vi "FaulhaberCommunication.vi"(7 "axis-optional-1":i16=-1, 8 "error in (no error)":errorcluster, 9 "Argument-optional":dbl=nan, 10 "Befehl":string="GAC", 11 "VISA resource name":refnum<visa-resource-name>="COM10") -> (0 "error out":errorcluster={"status"=FALSE, "code"=1073676293, "source"="VISA Read in FaulhaberCommunication.vi->Faulhaber_Standalone.vi"}, 1 "return":dbl, 2 "return":string="5000\r\n", 3 "VISA resource name out":refnum<visa-resource-name>="COM10")   [LabVIEW 2011]
uses:
  <vilib>/Instr/_visa.llb/VISA Flush IO Buffer Mask.ctl
panel:
  out "return count":u32=6
  in  "Array":T1(array[cluster])
  out "expect return":T2(ring)=enum."somethingelse16"
  out "to send unsigned byte array":u8[](array[numeric])=[71, 65, 67, 13] format="%02x"
  out "send":u32=4
  # "send ist CR\nZwischen befehl und Argument kein leerzeichen\nArgument bis I32\nantwort ist CR-LF"
  # "Gibt binär return:"
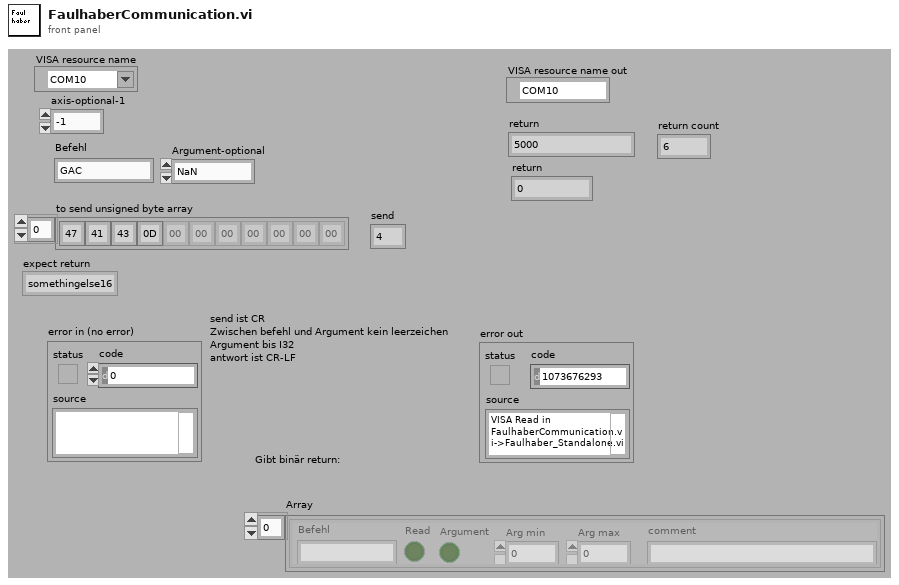
[diagram p1: front panel]
types:
  T1 = cluster{"Befehl":string, "Read":bool, "Arg min":dbl, "Arg max":dbl, "Argument":bool, "comment":string}[]
  T2 = enum8{"none", "program32", "program16", "data32", "data16", "eprom32", "eprom16", "somethingelse32", "somethingelse16"}
  T3 = typedef "VISA Flush IO Buffer Mask.ctl" = u16
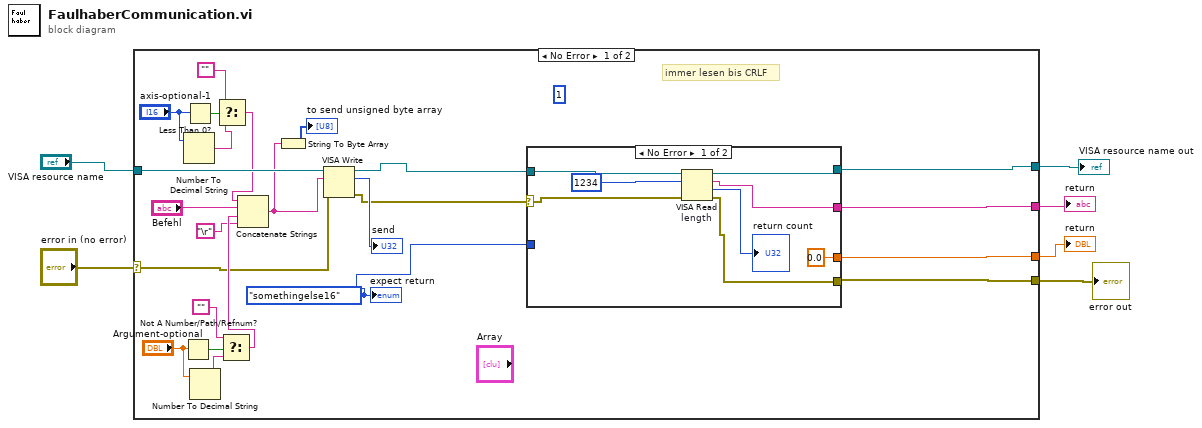
[diagram p0: block diagram]
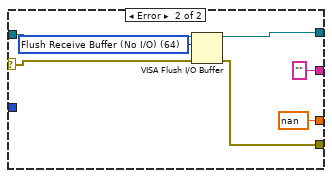
[diagram p2: hidden frame]
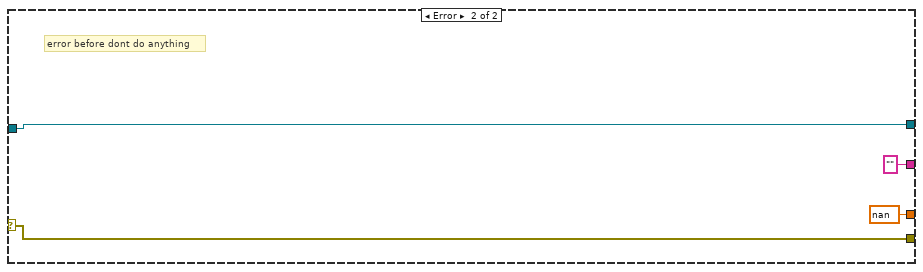
[diagram p3: hidden frame]
diagram:
  n1 = case shown="No Error" "error in (no error)" {
    selector: "error in (no error)" -> [w12 w48]
    tunnel: "VISA resource name" -> [w30 w49]
    tunnel: [w28 w49] -> w5
    tunnel: [w27 w48] -> w4
    tunnel: [w26 nan ("(hi.lo)")] -> w3
    tunnel: [w25 "" ("name")] -> w1
    frame No Error {
      (unwired) u32 1 ("byte count")
      w11 = T2."somethingelse16" ("expect return")
      # "immer lesen bis CRLF"
      n2 = Not A Number/Path/Refnum?(number/path/refnum="Argument-optional") -> (NaN/Path/Refnum?=w19:bool)
      n3 = Number To Decimal String(number="axis-optional-1") -> (decimal integer string=w22:string)  [unwired: 1 in]
      n4 = Less Than 0?(x="axis-optional-1") -> (x < 0?=w24:bool)
      n5 = Number To Decimal String(number="Argument-optional") -> (decimal integer string=w17:string)  [unwired: 1 in]
      n6 = Select(t="", s=w24, f=w22) -> (s? t:f=w16:string)
      n7 = Select(t="", s=w19, f=w17) -> (s? t:f=w14:string)
      n8 = Concatenate Strings(w16, "Befehl", w14, "\r") -> (w9:string)
      n9 = String To Byte Array(string=w9) -> (unsigned byte array=→"to send unsigned byte array":u8[])
      n10 = VISA Write(VISA resource name=w30, write buffer=w9, error in (no error)=w12) -> (VISA resource name out=w7:refnum<visa-resource-name>, return count=→"send":u32, error out=w8:errorcluster)
      n11 = case shown="No Error" w8 {
        selector: w8 -> [w36 w43]
        tunnel: w7 -> [w38 w45]
        tunnel: [w37 w44] -> w28
        tunnel: [w35 w42] -> w27
        tunnel: [0.0 ("(hi.lo)") nan ("(hi.lo)")] -> w26
        tunnel: [w34 "" ("read buffer")] -> w25
        tunnel: w11 -> [_ _]
        frame No Error {
          n12 = VISA Read "length"(VISA resource name=w38, byte count=u32 1234, error in (no error)=w36) -> (VISA resource name out=w37:refnum<visa-resource-name>, read buffer=w34:string, return count=→"return count":u32, error out=w35:errorcluster)
        }
        frame Error {
          w41 = T3 64 items=["Flush Receive Buffer"=16, "Write Transmit Buffer to Device"=32, "Flush Receive Buffer (No I/O)"=64, "Flush Transmit Buffer"=128] ("Mask")
          n13 = VISA Flush I/O Buffer(VISA resource name=w45, mask (16)=w41, error in (no error)=w43) -> (VISA resource name out=w44:refnum<visa-resource-name>, error out=w42:errorcluster)
        }
      }
      "expect return" <- w11
    }
    frame Error {
      # "error before dont do anything"
    }
  }
  "VISA resource name out" <- w5
  "error out" <- w4
  "return" <- w3
  "return" <- w1
